vi "Start Motive and PacketClient.vi"(8 "Error In":errorcluster) -> (0 "Error Out":errorcluster)   [LabVIEW 2017]
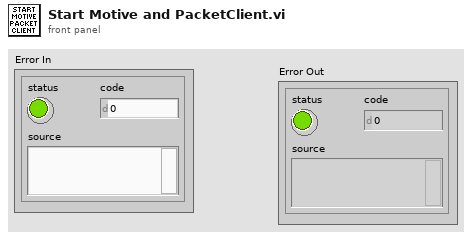
[diagram p1: front panel]
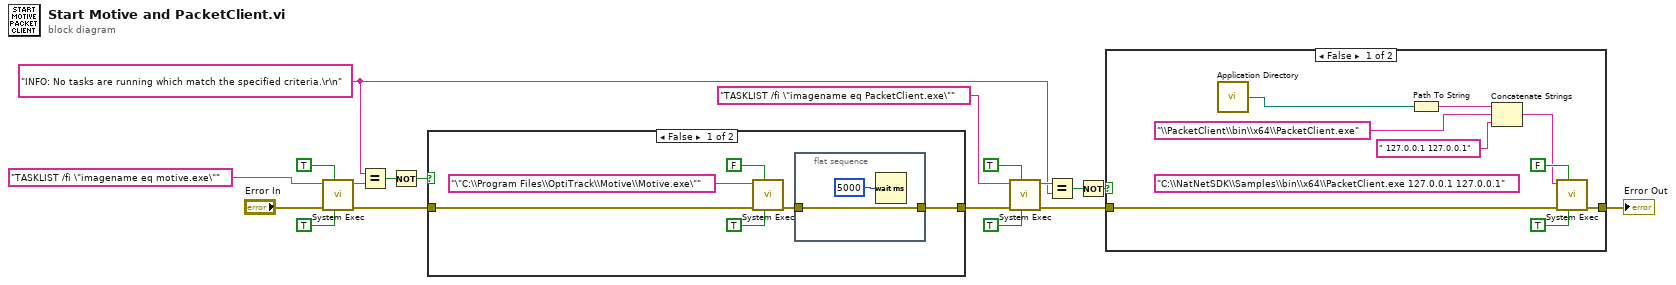
[diagram p0: block diagram]
diagram:
  w6 = "INFO: No tasks are running which match the specified criteria.\r\n" ("y")
  n1 = call <vilib>:"System Exec.vi"("run minimized? (F)"=TRUE, "wait until completion? (T)"=TRUE, "error in (no error)"="Error In", "command line"="TASKLIST /fi \"imagename eq motive.exe\"" ("String")) -> ("error out"=w9:errorcluster, "standard output"=w7:string)  [unwired: 4 in, 2 out]
  n2 = Equal?(x=w6, y=w7) -> (x = y?=w8:bool)
  n3 = Not(x=w8) -> (.not. x?=w5:bool)
  n4 = case shown="False" w5 {
    tunnel: [w21 w27] -> w2
    tunnel: w9 -> [w19 w27]
    frame False {
      n5 = call <vilib>:"System Exec.vi"("run minimized? (F)"=TRUE, "wait until completion? (T)"=FALSE, "error in (no error)"=w19, "command line"="\"C:\\Program Files\\OptiTrack\\Motive\\Motive.exe\"") -> ("error out"=w22:errorcluster)  [unwired: 4 in, 3 out]
      n6 = flat-sequence {
        tunnel: w22 -> [w25]
        tunnel: [w25] -> w21
        frame #0 {
          n7 = Wait (ms)(milliseconds to wait=u32 5000) -> ()  [unwired: 1 out]
        }
      }
    }
    frame True {
    }
  }
  n8 = call <vilib>:"System Exec.vi"("run minimized? (F)"=TRUE, "wait until completion? (T)"=TRUE, "error in (no error)"=w2, "command line"="TASKLIST /fi \"imagename eq PacketClient.exe\"" ("String")) -> ("error out"=w1:errorcluster, "standard output"=w17:string)  [unwired: 4 in, 2 out]
  n9 = Equal?(x=w17, y=w6) -> (x = y?=w16:bool)
  n10 = Not(x=w16) -> (.not. x?=w4:bool)
  n11 = case shown="False" w4 {
    tunnel: w1 -> [w34 w37]
    tunnel: [w33 w37] -> w3
    frame False {
      (unwired) "C:\\NatNetSDK\\Samples\\bin\\x64\\PacketClient.exe 127.0.0.1 127.0.0.1"
      n12 = call <vilib>:"Application Directory.vi"() -> ("Application Directory"=w29:path)
      n13 = Path To String(path=w29) -> (string=w32:string)
      n14 = Concatenate Strings(w32, "\\PacketClient\\bin\\x64\\PacketClient.exe" ("name or relative path"), " 127.0.0.1 127.0.0.1" ("string")) -> (w31:string)
      n15 = call <vilib>:"System Exec.vi"("run minimized? (F)"=TRUE, "wait until completion? (T)"=FALSE, "error in (no error)"=w34, "command line"=w31) -> ("error out"=w33:errorcluster)  [unwired: 4 in, 3 out]
    }
    frame True {
    }
  }
  "Error Out" <- w3
